vi "RM.initFPGADevice.vi"(8 "error in":errorcluster, 10 "device name":string="deviceName", 11 "Item Ref in":T1 format="%.0x") -> (0 "error out":errorcluster, 3 "Item Ref out":T1 format="%.0x")   [LabVIEW 2016, in "FPGA Addon Shared.lvlib"]
uses:
  FPGA Addon Shared.lvlib
  <vilib>/NI Veristand/Custom Device API/Custom Device Item Ref.ctl
  <vilib>/NI VeriStand/Custom Device API/Custom Device API.lvlib
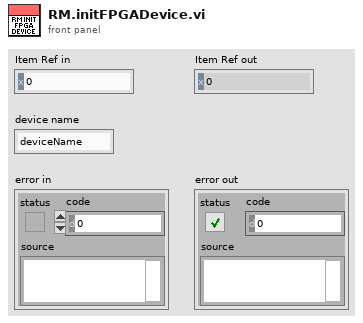
[diagram p1: front panel]
types:
  T1 = typedef "Custom Device API.lvlib/Custom Device Item Ref.ctl" = u64
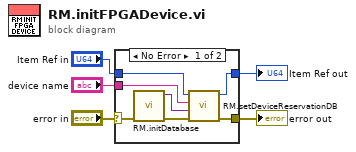
[diagram p0: block diagram]
diagram:
  n1 = case shown="No Error" "error in" {
    selector: "error in" -> [w7 w13]
    tunnel: "Item Ref in" -> [w12 w14]
    tunnel: [w11 w14] -> w4
    tunnel: "device name" -> [w10 _]
    tunnel: [w6 w13] -> w1
    frame No Error {
      n2 = call "RM.initDatabase.vi"("error in"=w7) -> ("error out"=w8:errorcluster, "reservation DB out"=w9:variant)  [unwired: 9 in]
      n3 = call "RM.setDeviceReservationDB.vi"("error in"=w8, "reservation DB in"=w9, "device name"=w10, "Item Ref in"=w12) -> ("error out"=w6:errorcluster, "Item Ref out"=w11:T1)  [unwired: 5 in, 1 out]
    }
    frame Error {
    }
  }
  "error out" <- w1
  "Item Ref out" <- w4
